vi "Quit.vi"(5 "Ask":bool=TRUE, 6 "Operation":T1, 7 "Message (Quit Program?)":string="Quit Program?", 8 "Error In":errorcluster, 9 "Quit":bool, 10 "F button name (\"Cancel\")":string="Cancel", 11 "T button name (\"OK\")":string="OK") -> (0 "Error Out":errorcluster, 1 "Quit?":bool)   [LabVIEW 2019]
uses:
  Utilities/Set_Read_Clear.ctl
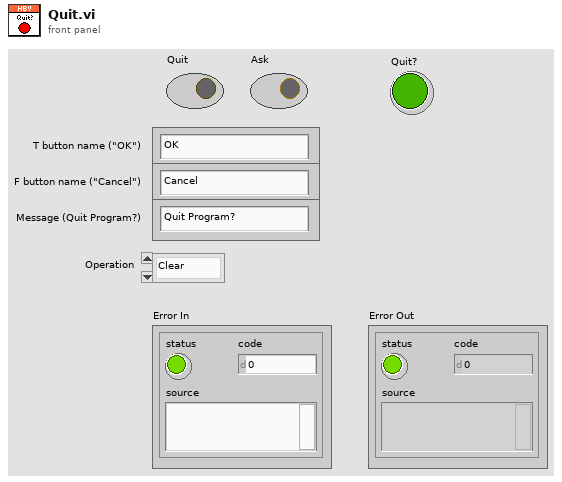
[diagram p1: front panel]
types:
  T1 = typedef "Set_Read_Clear.ctl" = enum16{"Clear", "Set", "Read"}
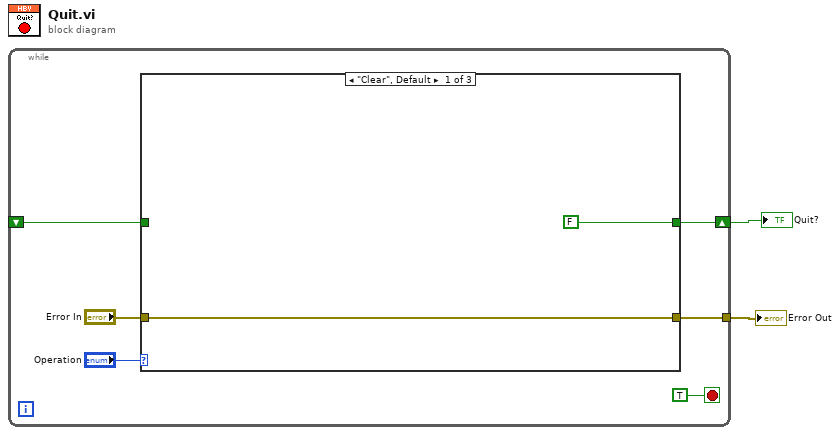
[diagram p0: block diagram]
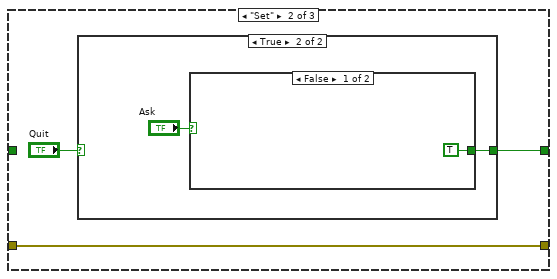
[diagram p2: hidden frame]
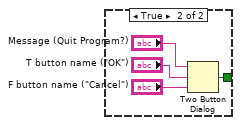
[diagram p4: hidden frame]
diagram:
  n1 = while {
    shift-right: [w7] -> w2
    shift-left: _ -> [w6]
    tunnel: [w3] -> w1
    stop <- TRUE stop-if-true
    n2 = case shown="\"Clear\", Default" "Operation" {
      tunnel: [FALSE ("T button?") w13 w23] -> w7
      tunnel: w6 -> [_ _ w23]
      tunnel: "Error In" -> [w9 w11 w22]
      tunnel: [w9 w11 w22] -> w3
      frame "Clear", Default {
      }
      frame "Set" {
        n3 = case shown="True" "Quit" {
          selector: "Quit" -> [w14 _]
          tunnel: [w14 w16] -> w13
          frame False {
          }
          frame True {
            n4 = case shown="False" "Ask" {
              tunnel: [TRUE ("T button?") w21] -> w16
              frame False {
              }
              frame True {
                n5 = Two Button Dialog(message="Message (Quit Program?)", 1:"F button name (\"Cancel\")", 2:"T button name (\"OK\")") -> (T button?=w21:bool)
              }
            }
          }
        }
      }
      frame "Read" {
      }
    }
  }
  "Error Out" <- w1
  "Quit?" <- w2
